vi "InvKinematicsCore.vi"(8 "Speed Constraints":T3, 9 "Speed Cap":dbl=1.0 format="%#_13g", 10 "Joystick Data":cluster{"X":dbl, "Y":dbl, "Z":dbl}, 11 "Pod Coordinates":cluster{"X":dbl, "Y":dbl}[](array[cluster])) -> (1 "Resultant Vector":T1, 2 "Pod User Data Out":T2(array[cluster]), 3 "Pod Plot Data Out":T4(array[cluster]))   [LabVIEW 2014]
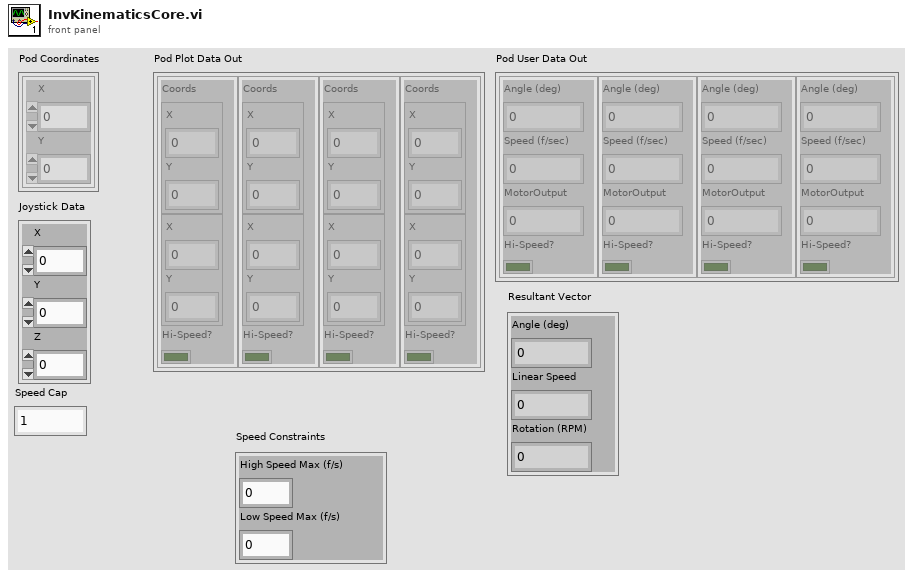
[diagram p1: front panel]
types:
  T1 = cluster{"Angle (deg)":dbl, "Linear Speed":dbl, "Rotation (RPM)":dbl}
  T2 = cluster{"Angle (deg)":dbl, "Speed (f/sec)":dbl, "MotorOutput":dbl, "Hi-Speed?":bool}[]
  T3 = cluster{"High Speed Max (f/s)":dbl, "Low Speed Max (f/s)":dbl}
  T4 = cluster{"Coords":cluster{"X":dbl, "Y":dbl}, "Vector":cluster{"X":dbl, "Y":dbl}, "Hi-Speed?":bool}[]
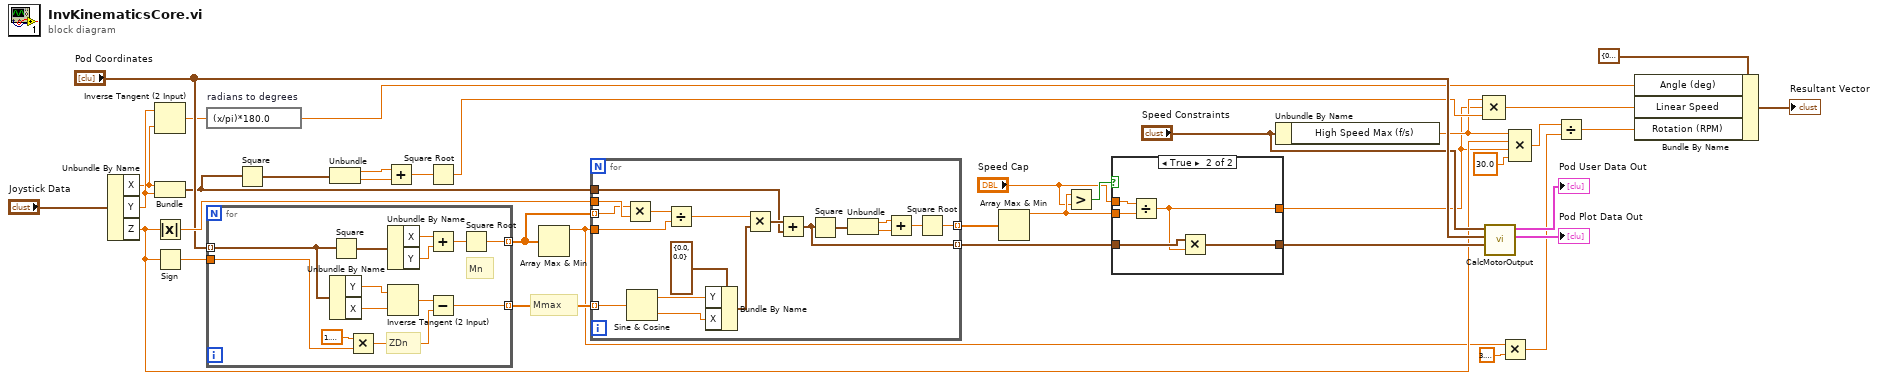
[diagram p0: block diagram]
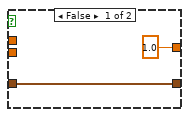
[diagram p2: hidden frame]
diagram:
  # "Mmax"
  n1 = Unbundle By Name("Joystick Data") -> ("X"=w17:dbl, "Y"=w18:dbl, "Z"=w8:dbl)
  n2 = Inverse Tangent (2 Input)(1:w17, 2:w18) -> (0:w21:dbl)
  n3 = Bundle("X"=w17, "Y"=w18) -> (w16:cluster{"X":dbl, "Y":dbl})  [unwired: 1 in]
  n4 = Absolute Value(x=w8) -> (abs(x)=w36:dbl)
  n5 = Sign(1:w8) -> (0:w29:dbl)
  n6 = expression code="(x/pi)*180.0" "radians to degrees"(w21) -> (w20:dbl)
  n7 = for {
    tunnel: "Pod Coordinates" -> [w40] mode=indexing
    tunnel: w29 -> [w48]
    tunnel: [w44] -> w31 mode=indexing
    tunnel: [w43] -> w30 mode=indexing
    # "ZDn"
    # "Mn"
    n8 = Unbundle By Name(w40) -> ("Y"=w39:dbl, "X"=w38:dbl)
    n9 = Square(x=w40) -> (x^2=w41:cluster{"X":dbl, "Y":dbl})
    n10 = Multiply(x=1.5707963267948966, y=w48) -> (x*y=w45:dbl)
    n11 = Unbundle By Name(w41) -> ("X"=w49:dbl, "Y"=w50:dbl)
    n12 = Inverse Tangent (2 Input)(1:w38, 2:w39) -> (0:w46:dbl)
    n13 = Add(x=w49, y=w50) -> (x+y=w42:dbl)
    n14 = Subtract(x=w46, y=w45) -> (x-y=w43:dbl)
    n15 = Square Root(x=w42) -> (sqrt(x)=w44:dbl)
  }
  n16 = Square(x=w16) -> (x^2=w15:cluster{"X":dbl, "Y":dbl})
  n17 = Unbundle(w15) -> ("X"=w13:dbl, "Y"=w14:dbl)
  n18 = Add(x=w13, y=w14) -> (x+y=w12:dbl)
  n19 = Square Root(x=w12) -> (sqrt(x)=w11:dbl)
  n20 = Array Max & Min(array=w31) -> (max value=w3:dbl)  [unwired: 3 out]
  n21 = for {
    tunnel: w30 -> [w64] mode=indexing
    tunnel: w31 -> [w67] mode=indexing
    tunnel: w3 -> [w65]
    tunnel: w36 -> [w68]
    tunnel: w16 -> [w58]
    tunnel: [w54] -> w34 mode=indexing
    tunnel: [w55] -> w32 mode=indexing
    n22 = Multiply(x=w67, y=w68) -> (x*y=w66:dbl)
    n23 = Sine & Cosine(0:w64) -> (1:w62:dbl, 2:w61:dbl)
    n24 = Divide(x=w66, y=w65) -> (x/y=w60:dbl)
    n25 = Bundle By Name(cluster=cluster{"X":dbl, "Y":dbl} {"X"=0.0, "Y"=0.0} ("Axes"), "Y"=w62, "X"=w61) -> (w51:cluster{"X":dbl, "Y":dbl})
    n26 = Multiply(x=w60, y=w51) -> (x*y=w59:cluster{"X":dbl, "Y":dbl})
    n27 = Add(x=w59, y=w58) -> (x+y=w54:cluster{"X":dbl, "Y":dbl})
    n28 = Square(x=w54) -> (x^2=w53:cluster{"X":dbl, "Y":dbl})
    n29 = Unbundle(w53) -> ("X"=w56:dbl, "Y"=w57:dbl)
    n30 = Add(x=w56, y=w57) -> (x+y=w52:dbl)
    n31 = Square Root(x=w52) -> (sqrt(x)=w55:dbl)
  }
  n32 = Array Max & Min(array=w32) -> (max value=w35:dbl)  [unwired: 3 out]
  n33 = Greater?(x=w35, y="Speed Cap") -> (0:w33:bool)
  n34 = case shown="True" w33 {
    tunnel: w34 -> [w70 w73]
    tunnel: w35 -> [_ w74]
    tunnel: [w70 w72] -> w26
    tunnel: "Speed Cap" -> [_ w75]
    tunnel: [1.0 w71] -> w7
    frame False {
    }
    frame True {
      n35 = Divide(x=w75, y=w74) -> (x/y=w71:dbl)
      n36 = Multiply(x=w73, y=w71) -> (x*y=w72:cluster{"X":dbl, "Y":dbl}[])
    }
  }
  n37 = Unbundle By Name("Speed Constraints") -> ("High Speed Max (f/s)"=w9:dbl)
  n38 = Compound Arithmetic op=MULTIPLY(w9, w7, w11) -> (w10:dbl)
  n39 = call "CalcMotorOutput.vi"("Pod Vectors"=w26, "Pod Coordinates"="Pod Coordinates", "Speed Constraints"="Speed Constraints") -> ("Pod Plot Data Out"=→"Pod Plot Data Out":T4, "Pod User Data Out"=→"Pod User Data Out":T2)  [unwired: 7 in]
  n40 = Multiply(x=w3, y=3.141592653589793) -> (x*y=w4:dbl)
  n41 = Compound Arithmetic op=MULTIPLY(w9, w8, w7, 30.0 ("value")) -> (w5:dbl)
  n42 = Divide(x=w5, y=w4) -> (x/y=w1:dbl)
  n43 = Bundle By Name(cluster=T1 {"Angle (deg)"=0.0, "Linear Speed"=0.0, "Rotation (RPM)"=0.0} ("Resultant Vector"), "Angle (deg)"=w20, "Linear Speed"=w10, "Rotation (RPM)"=w1) -> (→"Resultant Vector":T1)
